vi "LNA Return Message.vi"(8 "Error In":errorcluster, 10 "LNA Return Message Msg":refnum<class "LNA Return Message Msg.lvclass">, 11 "TestLNA in":refnum<class "TestLNA.lvclass">) -> (0 "Error Out":errorcluster, 3 "TestLNA out":refnum<class "TestLNA.lvclass">)   [LabVIEW 2014, in "TestLNA.lvlib" / "TestLNA.lvclass"]
uses:
  TestLNA.lvclass
  LNA Messages/LNA Return Message Msg/LNA Return Message Msg.lvclass
  CSPP_Core/Actors/CS++BaseActor/CS++BaseActor.lvclass/CS++BaseActor.ctl
  CSPP_Core/Actors/CS++BaseActor/Read Object Name.vi
  <vilib>/NI/Actors/Linked Network Actor/Linked Network Actor Messages/LNA Return Message Msg/LNA Return Message Msg.lvclass
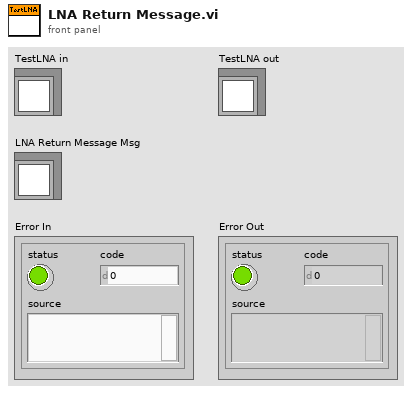
[diagram p1: front panel]
types:
  T1 = typedef "Actor Framework.lvlib/Message Enqueuer.lvclass/Message Priority.ctl" = enum16{"Low", "Normal", "High"}
  T2 = cluster{"Tx Message":refnum<class "Message.lvclass">, "Tx Error":errorcluster, "Message Priority":T1}
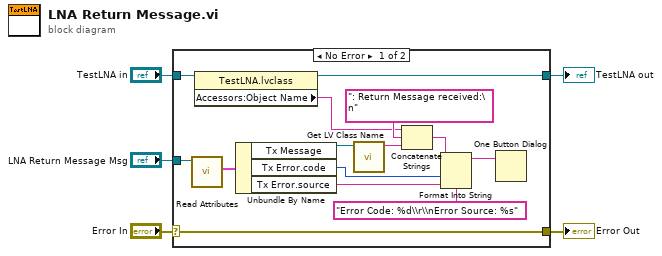
[diagram p0: block diagram]
diagram:
  n1 = case shown="No Error" "Error In" {
    selector: "Error In" -> [w18 w21]
    tunnel: [w18 w21] -> w4
    tunnel: [w7 w20] -> w2
    tunnel: "TestLNA in" -> [w19 w20]
    tunnel: "LNA Return Message Msg" -> [w9 _]
    frame No Error {
      n2 = call <vilib>:"Read Attributes.vi"("Abstract Message Template in"=w9) -> ("Payload"=w17:T2)  [unwired: 9 in, 1 out]
      n3 = property class="TestLNA.lvclass"(reference=w19) -> (reference out=w7:refnum<class "TestLNA.lvclass">, "Accessors:Object Name"=w6:string)  [unwired: 1 in, 1 out]
      n4 = Unbundle By Name(w17) -> ("Tx Message"=w16:refnum<class "Message.lvclass">, "Tx Error.code"=w12:i32, "Tx Error.source"=w11:string)
      n5 = call <vilib>:"Get LV Class Name.vi"("object"=w16) -> ("class name"=w15:string)  [unwired: 9 in, 1 out]
      n6 = Concatenate Strings(w6, ": Return Message received:\n", w15) -> (w14:string)
      n7 = Format Into String(format string="Error Code: %d\\r\\nError Source: %s", initial string=w14, w12, w11) -> (resulting string=w13:string)  [unwired: 1 in, 1 out]
      n8 = One Button Dialog(message=w13) -> ()  [unwired: 1 in, 1 out]
    }
    frame Error {
    }
  }
  "Error Out" <- w4
  "TestLNA out" <- w2
